vi "Restore AO Amplitudes.vi"(8 "error in (no error)":errorcluster, 10 "Saved Amplitudes":dbl[](array[numeric]), 11 "Instrument.DAQ in":refnum<class "Instrument.DAQ.lvclass">) -> (0 "error out":errorcluster, 3 "Instrument.DAQ out":refnum<class "Instrument.DAQ.lvclass">)   [LabVIEW 2019, in "Instrument.Lockin.lvlib" / "Instrument.DAQ.lvclass"]
uses:
  Instrument.DAQ.lvclass
  Instrument.DAQ.lvclass/Instrument.DAQ.ctl
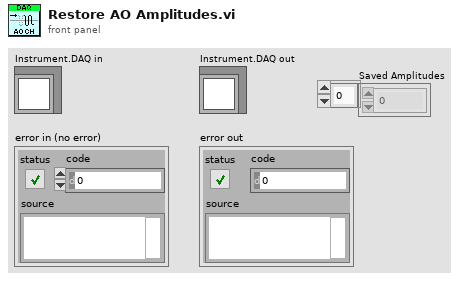
[diagram p1: front panel]
types:
  T1 = typedef "Instrument.Lockin.lvlib/Instrument.DAQ.lvclass/AO.Channel--Cluster--Array.ctl" = T2[]
  T2 = typedef "Instrument.Lockin.lvlib/Instrument.DAQ.lvclass/AO.Channel--Cluster.ctl" = cluster{"Enable?":bool, "Channel":i32, "Amplitude":dbl, "Offset":dbl, "Frequency":dbl, "Phase":dbl, "Function":T3, "Sweeping?":bool, "Limit AC":bool, "Limit DC?":bool, "Duty Cycle":bool}
  T3 = typedef "Instrument.Lockin.lvlib/Instrument.DAQ.lvclass/AO.Channel.Function--Enum.ctl" = enum16{"sine", "square", "triangle", "saw"}
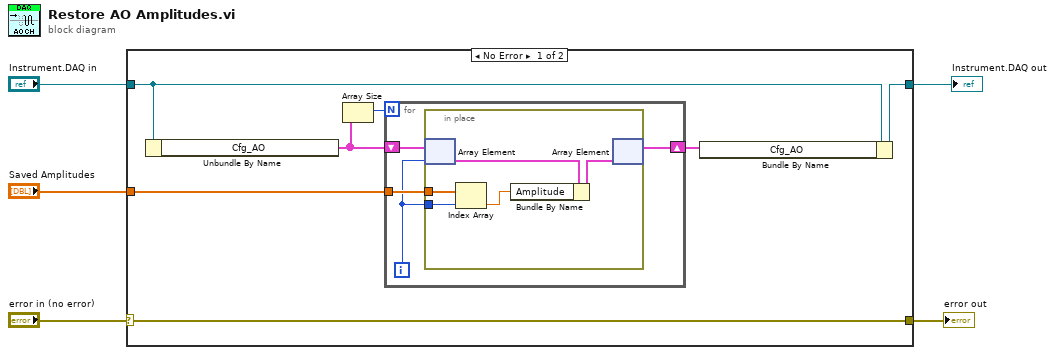
[diagram p0: block diagram]
diagram:
  n1 = case shown="No Error" "error in (no error)" {
    selector: "error in (no error)" -> [w7 w23]
    tunnel: [w11 w22] -> w5
    tunnel: "Instrument.DAQ in" -> [w10 w22]
    tunnel: [w7 w23] -> w2
    tunnel: "Saved Amplitudes" -> [w6 _]
    frame No Error {
      n2 = Unbundle By Name(w10) -> ("Cfg_AO"=w9:T1)
      n3 = Array Size(array=w9) -> (size(s)=w8:i32)
      n4 = for {
        N: w8 -> [_]
        shift-right: [w15] -> w12
        shift-left: w9 -> [w16]
        tunnel: w6 -> [w14]
        i -> [w13]
        n5 = in-place {
          in-place-border: w14 -> [w18]
          in-place-border: w13 -> [w19]
          n6 = in-place-array #1(w16, w13) -> (w21:T2)
          n7 = Index Array(array=w18, index=w19) -> (element=w17:dbl)
          n8 = Bundle By Name(cluster=w21, "Amplitude"=w17) -> (w20:T2)
          n9 = in-place-array #1(w20) -> (w15:T1)  [unwired: 1 out]
        }
      }
      n10 = Bundle By Name(cluster=w10, "Cfg_AO"=w12) -> (w11:refnum<class "Instrument.DAQ.lvclass">)
    }
    frame Error {
    }
  }
  "error out" <- w2
  "Instrument.DAQ out" <- w5
